vi "Write Char Data to S1P.vi"(0 "VISA resource name":refnum<visa-resource-name>, 1 "S1P File Path In":path, 5 "ACM Path":T2, 7 "S-Parameter":T1, 11 "error in (no error)":errorcluster) -> (3 "S1P File Path Out":path, 4 "VISA resource name out":refnum<visa-resource-name>, 15 "error out":errorcluster)   [LabVIEW 2023, in "ACM Visa Driver.lvlib"]
uses:
  ACM Visa Driver.lvlib
  API/Controls/ACM Paths.ctl
  API/Controls/ACM S-Parameters.ctl
  HFNetworkAnalysis/Controls/SnPDataType.ctl
  HFNetworkAnalysis/NI_HFNetworkAnalysis.lvlib
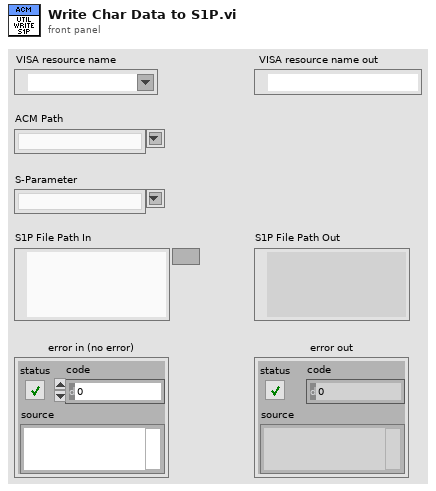
[diagram p1: front panel]
types:
  T1 = typedef "ACM Visa Driver.lvlib/ACM S-Parameters.ctl" = string
  T2 = typedef "ACM Visa Driver.lvlib/ACM Paths.ctl" = string
  T3 = typedef "NI_HFNetworkAnalysis.lvlib/SnPDataType.ctl" = enum16{"DB", "MA", "RI"}
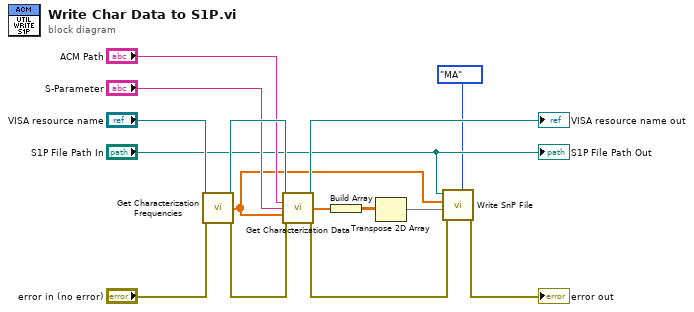
[diagram p0: block diagram]
diagram:
  n1 = call "Get Characterization Frequencies.vi"("VISA resource name"="VISA resource name", "error in (no error)"="error in (no error)") -> ("VISA resource name out"=w15:refnum<visa-resource-name>, "S-Par Characterization Frequencies"=w2:dbl[], "error out"=w14:errorcluster)  [unwired: 11 in]
  n2 = call "Get Characterization Data.vi"("VISA resource name"=w15, "ACM Path"="ACM Path", "S-Parameter"="S-Parameter", "Characterization Frequencies (for Temp Co)"=w2, "error in (no error)"=w14) -> ("VISA resource name out"=→"VISA resource name out":refnum<visa-resource-name>, "S-Par Characterization Data"=w5:cdb[], "error out"=w11:errorcluster)  [unwired: 8 in]
  n3 = Build Array(w5) -> (w3:cdb[][])
  n4 = Transpose 2D Array(2D array=w3) -> (transposed array=w4:cdb[][])
  n5 = call "Write SnP File.vi"("OutputDataType"=SnPDataType."MA", "error in (no error)"=w11, "S-parameters"=w4, "Frequencies (Hz)"=w2, "SnP File Path"="S1P File Path In") -> ("error out"=→"error out":errorcluster)  [unwired: 6 in]
  "S1P File Path Out" <- "S1P File Path In"
